vi "ReadSymbolProperties.vi"(8 "error in (no error)":errorcluster, 11 "AdsNET in":refnum<class "AdsNET.lvclass">) -> (0 "error out":errorcluster, 2 "SymbolProperties":T1(array[cluster]), 3 "AdsNET out":refnum<class "AdsNET.lvclass">)   [LabVIEW 2016, in "TCatAdsNet.lvlib" / "AdsNET.lvclass"]
uses:
  AdsNET.lvclass
  AdsNET.lvclass/AdsNET.ctl
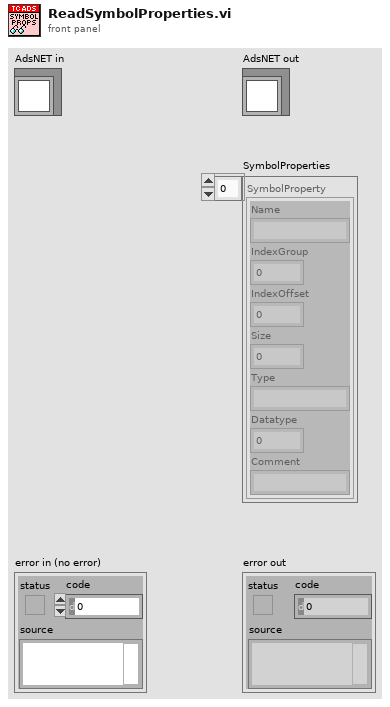
[diagram p1: front panel]
types:
  T1 = cluster{"Name":string, "IndexGroup":i64, "IndexOffset":i64, "Size":i32, "Type":string, "Datatype":i32, "Comment":string}[]
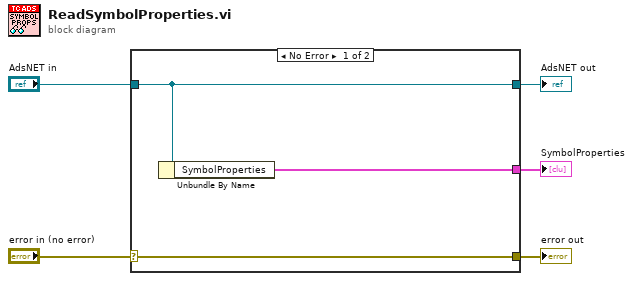
[diagram p0: block diagram]
diagram:
  n1 = case shown="No Error" "error in (no error)" {
    selector: "error in (no error)" -> [w8 w9]
    tunnel: [w8 w9] -> w4
    tunnel: [w7 w10] -> w2
    tunnel: "AdsNET in" -> [w7 w10]
    tunnel: [w6 _] -> w1
    frame No Error {
      n2 = Unbundle By Name(w7) -> ("SymbolProperties"=w6:T1)
    }
    frame Error {
    }
  }
  "error out" <- w4
  "AdsNET out" <- w2
  "SymbolProperties" <- w1
